vi "camara.vi"() -> ()   [LabVIEW 2010]
uses:
  <vilib>/addons/PixeLINK/Low Level Functions/CAMERA_FEATURES.llb/TDPU-CameraFeatures-PixelFormat.ctl
  <vilib>/vision/Image Controls.llb/IMAQ Image.ctl
  <vilib>/vision/NI_Vision_Development_Module.lvlib
panel:
  in  "First Call?: T/F":bool
  out "Line Profile":dbl[](graph)
  out "Gray Level Intensities":T1 {"Standard  Deviation" format="%.2f"; "Mean Intensity" format="%.2f"; "Maximum Intensity" format="%.2f"; "Minimum Intensity" format="%.2f"}
  in  "Boolean":bool
  out "time(ms)":u32
  in  "Tab Control":enum32{"Camara"}(tab)
  in  "Selector":u16(ring) items=["776002034"]
  in  "Streeam?":bool
  out "Camara Funciona?":bool
  out "Contraste":dbl(graph)
  out "Image":T2(plugin-control)
  in  "Grabar":bool
  in  "Camera Parameters":T4 {"Pixel Format" items=["PIXEL_FORMAT_MONO8", "PIXEL_FORMAT_MONO16", "PIXEL_FORMAT_YUV422", "PIXEL_FORMAT_BAYER8_GRBG", "PIXEL_FORMAT_BAYER16_GRBG", "PIXEL_FORMAT_RGB24", "PIXEL_FORMAT_RGB48", "PIXEL_FORMAT_BAYER8_RGGB", "PIXEL_FORMAT_BAYER8_GBRG ", "PIXEL_FORMAT_BAYER8_BGGR ", "PIXEL_FORMAT_BAYER16_RGGB ", "PIXEL_FORMAT_BAYER16_GBRG", "PIXEL_FORMAT_BAYER16_BGGR", "PIXEL_FORMAT_RGB32"]}
  in  "stop":bool
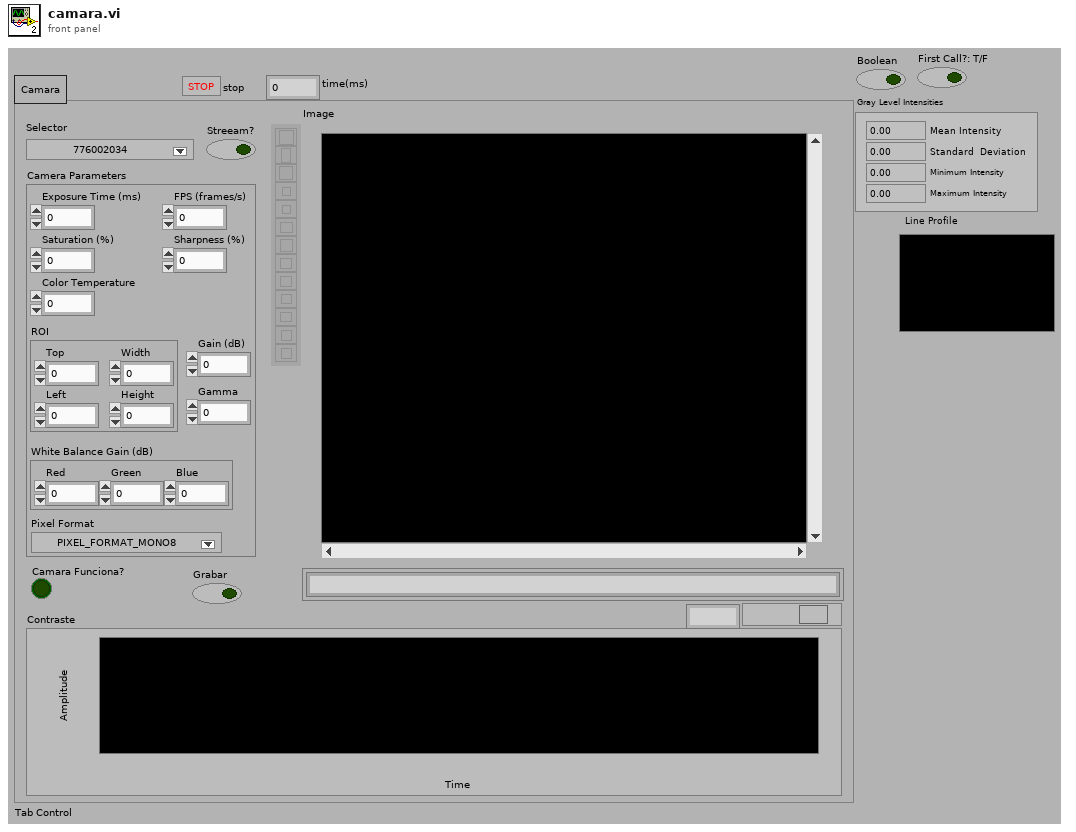
[diagram p1: front panel]
types:
  T1 = cluster{"Mean Intensity":sgl, "Standard  Deviation":sgl, "Minimum Intensity":sgl, "Maximum Intensity":sgl}
  T2 = typedef "IMAQ Image.ctl" = refnum<image>
  T3 = typedef "TDPU-CameraFeatures-PixelFormat.ctl" = u16
  T4 = cluster{"Exposure Time (ms)":dbl, "Gain (dB)":dbl, "Saturation (%)":dbl, "Sharpness (%)":dbl, "Color Temperature":dbl, "ROI":cluster{"Top":i32, "Left":i32, "Width":i32, "Height":i32}, "White Balance Gain (dB)":cluster{"Red":dbl, "Green":dbl, "Blue":dbl}, "Gamma":dbl, "Pixel Format":T3, "FPS (frames/s)":i32}
  T5 = cluster{"hCamera":u32, "Error":errorcluster, "uSerialNumber OUT":u32}
  T6 = cluster{"hCamera":u32, "Error":errorcluster, "uSerialNumber":u32}
  T7 = typedef "Image Type" = u32
  T8 = typedef "IMAQ Line" = cluster{"Start X":i32, "Start Y":i32, "End X":i32, "End Y":i32}
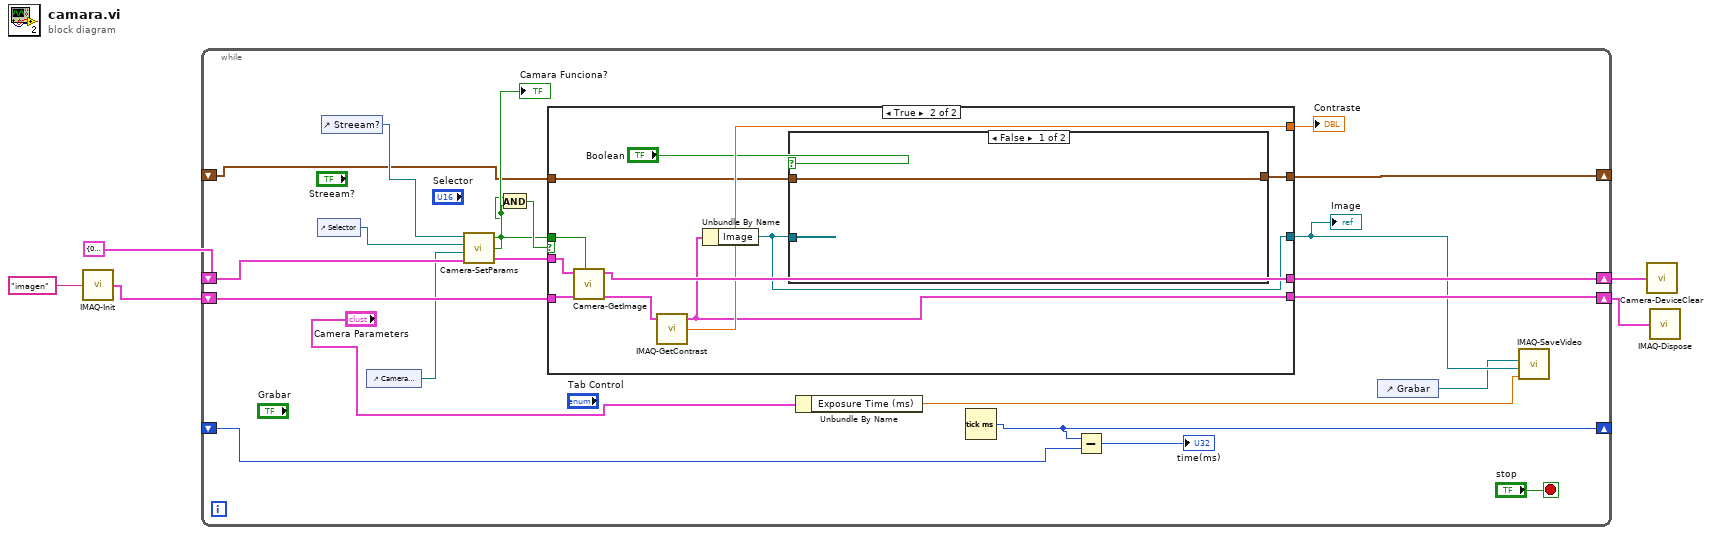
[diagram p0: block diagram]
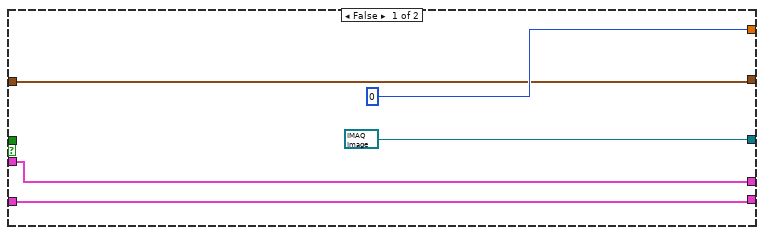
[diagram p2: hidden frame]
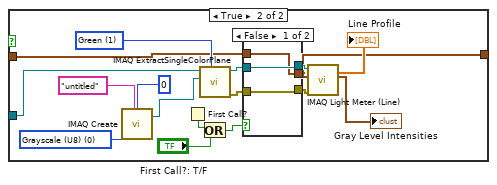
[diagram p3: hidden frame]
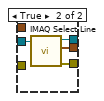
[diagram p4: hidden frame]
diagram:
  n1 = call "IMAQ-Init.vi"("Image Name"="imagen") -> ("Image Device IN"=w4:cluster{"Image":T2, "errorImage":errorcluster})
  n2 = while {
    shift-right: [w20] -> w1
    shift-left: w4 -> [w23]
    shift-right: [w22] -> w2
    shift-left: T5 {"hCamera"=0, "Error"={"status"=FALSE, "code"=0, "source"=""}, "uSerialNumber OUT"=0} ("Camera Device  IN") -> [w21]
    shift-right: [w13] -> _
    shift-left: _ -> [w12]
    shift-right: [w7] -> _
    shift-left: _ -> [w6]
    stop <- "stop" stop-if-true
    n3 = control-ref of="Selector"() -> (w26:refnum<vi>)
    n4 = control-ref of="Streeam?"() -> (w25:refnum<vi>)
    n5 = control-ref of="Camera Parameters"() -> (w8:refnum<vi>)
    n6 = call "Camera-SetParams.vi"("Camera Device  IN"=w21, "Camera Parameters"=w8, "Selector"=w26, "Stream?"=w25) -> ("Camera Device OUT"=w24:T6, "Funciona?"=w18:bool, "Stream? OUT"=w17:bool)
    "Camara Funciona?" <- w18
    n7 = And(x=w17, y=w18) -> (x .and. y?=w19:bool)
    n8 = case shown="True" w19 {
      tunnel: w24 -> [w32 w42]
      tunnel: w17 -> [_ w43]
      tunnel: w23 -> [w31 w41]
      tunnel: [w32 w40] -> w22
      tunnel: [T2 refnum ("Image") w33] -> w14
      tunnel: [w31 w37] -> w20
      tunnel: [u32 0 ("Numeric") w39] -> w16
      tunnel: [w28 w35] -> w7
      tunnel: w6 -> [w28 w34]
      frame False {
      }
      frame True {
        n9 = call "Camera-GetImage.vi"("Streeam"=w43, "Image Device IN"=w41, "Camera Device IN"=w42) -> ("Image Device OUT"=w38:cluster{"Image":T2, "errorImage":errorcluster}, "Camera Device OUT"=w40:T6)  [unwired: 4 in]
        n10 = call "IMAQ-GetContrast.vi"("Image Device IN"=w38) -> ("RMS Contraste"=w39:dbl, "Image Device OUT"=w37:cluster{"Image":T2, "errorImage":errorcluster})  [unwired: 3 in]
        n11 = Unbundle By Name(w37) -> ("Image"=w33:T2)
        n12 = case shown="False" "Boolean" {
          tunnel: w33 -> [_ w47]
          tunnel: [w44 w50] -> w35
          tunnel: w34 -> [w44 w49]
          frame False {
          }
          frame True {
            w53 = T7 0 items=["Grayscale (U8)", "Grayscale (I16)", "Grayscale (SGL)", "Complex (CSG)", "RGB (U32)", "HSL (U32)", "RGB (U64)", "Grayscale (U16)"] ("Image Type")
            w61 = 1 items=["Red", "Green", "Blue", "Hue", "Saturation", "Luminance", "Value", "Intensity"] ("Color Plane")
            n13 = call "IMAQ Create"("Border Size"=0, "Image Name"="untitled", "Image Type"=w53) -> ("New Image"=w56:T2)  [unwired: 2 in, 1 out]
            n14 = First Call?() -> (First Call?: T/F=w45:bool)
            n15 = call "IMAQ ExtractSingleColorPlane"("Color Plane"=w61, "Image Dst"=w56, "Image Src"=w47) -> ("error out"=w51:errorcluster, "Image Dst Out"=w60:T2)  [unwired: 7 in]
            n16 = Or(x=w45, y="First Call?: T/F") -> (x .or. y?=w46:bool)
            n17 = case shown="False" w46 {
              tunnel: w60 -> [w64 w68]
              tunnel: [w63 w67] -> w59
              tunnel: [w62 w66] -> w50
              tunnel: [w64 w65] -> w58
              tunnel: w51 -> [w63 _]
              tunnel: w49 -> [w62 _]
              frame False {
              }
              frame True {
                n18 = call "IMAQ Select Line"("Image In"=w68) -> ("error out"=w67:errorcluster, "Line"=w66:T8, "Image Out (duplicate)"=w65:T2)  [unwired: 7 in, 1 out]
              }
            }
            n19 = call "IMAQ Light Meter (Line)"("error in (no error)"=w59, "Line"=w50, "Image"=w58) -> ("Gray Level Intensities"=→"Gray Level Intensities":T1, "Line Profile"=→"Line Profile":dbl[])  [unwired: 4 in, 3 out]
          }
        }
      }
    }
    "Image" <- w14
    "Contraste" <- w16
    n20 = Unbundle By Name("Camera Parameters") -> ("Exposure Time (ms)"=w15:dbl)
    n21 = Tick Count (ms)() -> (millisecond timer value=w13:u32)
    n22 = Subtract(x=w13, y=w12) -> (x-y=→"time(ms)":u32)
    n23 = control-ref of="Grabar"() -> (w10:refnum<vi>)
    n24 = call "IMAQ-SaveVideo.vi"("Exposure Time (ms)"=w15, "Image"=w14, "Grabar"=w10) -> ()  [unwired: 1 in, 1 out]
  }
  n25 = call "Camera-DeviceClear.vi"("Camera Device OUT"=w2) -> ()
  n26 = call "IMAQ-Dispose.vi"("Image Device IN"=w1) -> ()
